vi "Virtual Launch HMI.vi"(8 "error in (no error)":errorcluster caption="entrée d'erreur (pas d'erreur)", 11 "ID":string) -> (0 "error out":errorcluster caption="sortie d'erreur", 2 "Input":string, 3 "Operator_Selection":bool)   [LabVIEW 2020, in "Library Instrument & Equipement.lvlib" / "Library Popup.lvlib" / "Class Popup (Main).lvclass"]
uses:
  Class Popup (Main).lvclass
  Commun VI/Library Commun.lvlib
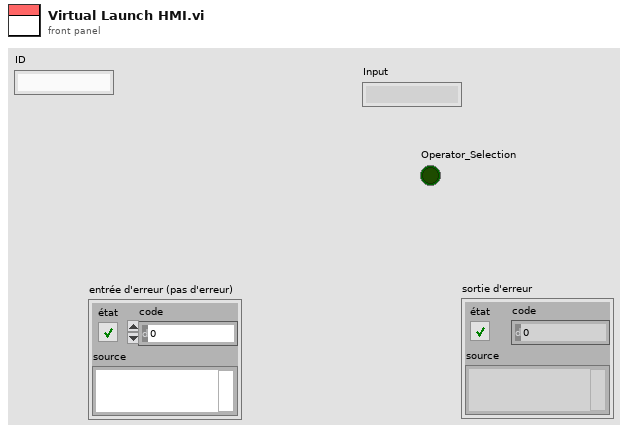
[diagram p1: front panel]
types:
  T1 = enum16{"Get Variable", "Get All Variables", "Set Variable", "Delete Variable", "Delete All Variable"}
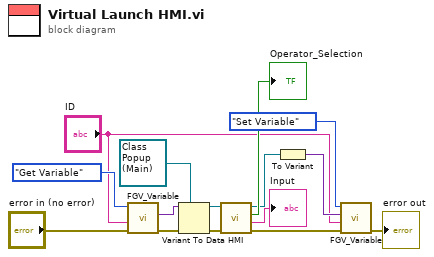
[diagram p0: block diagram]
diagram:
  n1 = call "FGV_Variable.vi"("error in (no error)"="error in (no error)", "Variable"="ID", "Function"=T1."Get Variable") -> ("error out"=w11:errorcluster, "Data Out"=w8:variant)  [unwired: 6 in, 1 out]
  n2 = Variant To Data(error in=w11, type=refnum<class "Class Popup (Main).lvclass"> refnum ("Class Popup (Main) en entrée"), Variant=w8) -> (data=w7:refnum<class "Class Popup (Main).lvclass">, error out=w10:errorcluster)
  n3 = call-dynamic "HMI.vi"("error in (no error)"=w10, "Class Popup (Main) en entrée"=w7) -> ("error out"=w2:errorcluster, "Input"=→"Input":string, "Operator_Selection"=→"Operator_Selection":bool, "Class Popup (Main) en sortie"=w4:refnum<class "Class Popup (Main).lvclass">)  [unwired: 6 in]
  n4 = To Variant(anything=w4) -> (Variant=w5:variant)
  n5 = call "FGV_Variable.vi"("error in (no error)"=w2, "Variable"="ID", "Data In"=w5, "Function"=T1."Set Variable") -> ("error out"=→"error out":errorcluster)  [unwired: 5 in, 2 out]
